vi "clm.build.flow.parse.vi"(11 "Device Flow":T1[](array[typedef])) -> (0 "error out":errorcluster, 3 "Device Conf":T3={"Schedular"={"sched-mode"=enum."Hourly", "sched-pairs"=[]}, "Sensor"={"Input"="ain", "Comparison"=">=", "Setpoint"=0.0}, "Outputs"=[], "Interval"=0, "Timeout"=0, "Mode"=enum."On"} caption="Device Setup" {"Schedular"."sched-pairs"."start" format="%<%H:%M %d/%m>T"; "Schedular"."sched-pairs"."stop" format="%<%H:%M %d/%m>T"; "Timeout" min=1})   [LabVIEW 2024]
uses:
  controls/UiStepBuilder.ctl
  controls/type.step-builder.ctl
  controls/controller.ctl
  controls/sched-cluster.ctl
  controls/UiScheduleTimestamp.ctl
  controls/UiDeviceSensorParams.ctl
  controls/UiDeviceSensorEquality.ctl
  controls/device-mode.ctl
  controls/sched-encoded-cluster.ctl
panel:
  out "length":i32
  out "Device Flow Out":T1[](array[typedef])=[{"Step Function"=enum."LOG-MESSAGE", "ParamString"="SENSOR", "Step Label"="DEVTYPE"}, {"Step Function"=enum."IO-COMPARE-OUT", "ParamString"="ain,>=,15.0,OFF,", "Step Label"="START"}, {"Step Function"=enum."IO-WRITE", "ParamString"="dout1,1:5", "Step Label"="ON"}, {"Step Function"=enum."JUMP", "ParamString"="WAIT", "Step Label"=""}, {"Step Function"=enum."IO-WRITE", "ParamString"="dout1,0:0", "Step Label"="OFF"}, {"Step Function"=enum."DELAY", "ParamString"="10", "Step Label"="WAIT"}, {"Step Function"=enum."JUMP", "ParamString"="START", "Step Label"=""}]
  # "Pulse [sec]"
  # "Period [sec]"
  # "Sensor"
  # "Scheduler"
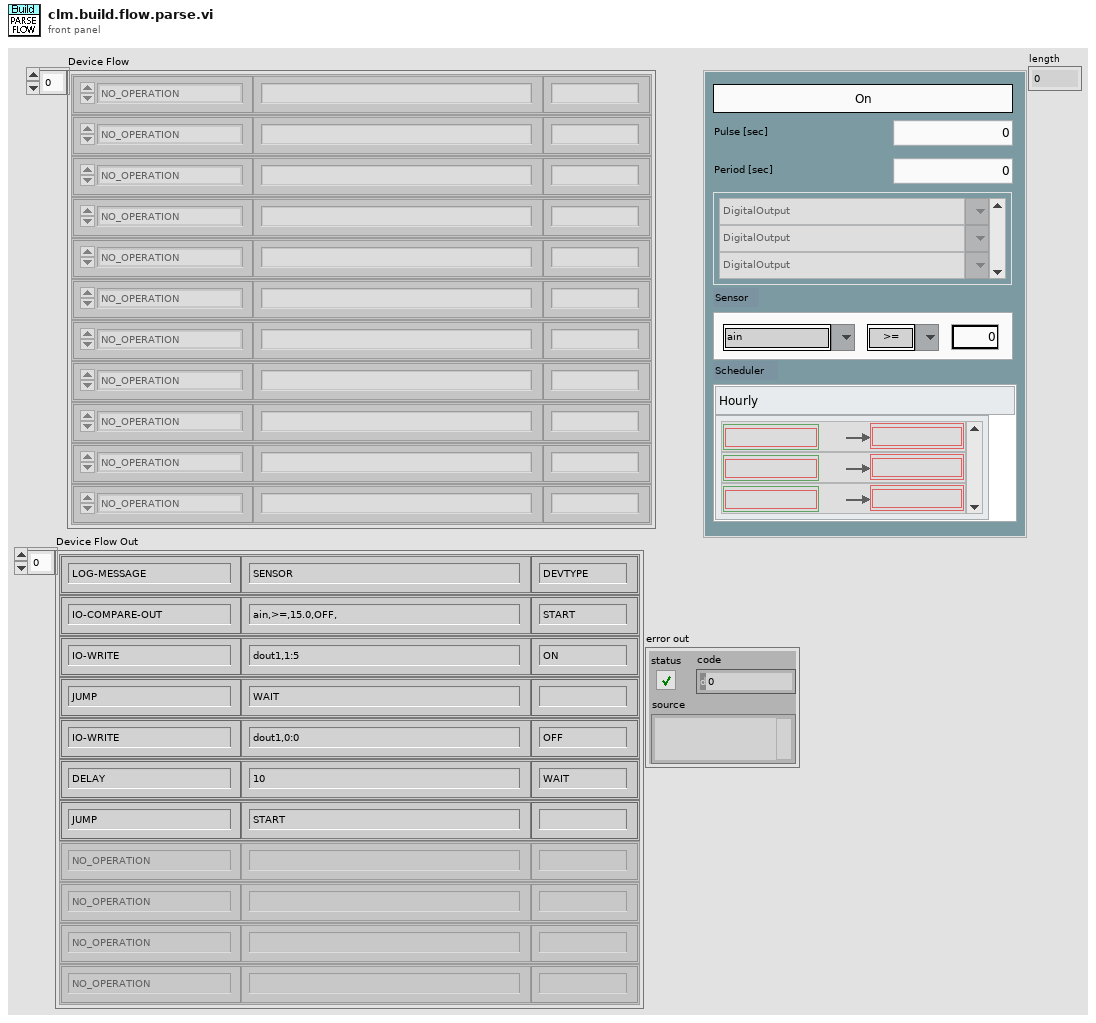
[diagram p1: front panel]
types:
  T1 = typedef "UiStepBuilder.ctl" = cluster{"Step Function":T2, "ParamString":string, "Step Label":string}
  T2 = typedef "type.step-builder.ctl" = enum16{"NO_OPERATION", "DELAY-JUMP", "DELAY", "JUMP", "COMPLETE", "SCHEDULER", "IRR-CHECK", "UNIT-CHECK", "UNIT-SAMPLE", "UNIT-DOSE", "LOG-REPORT", "LOG-MESSAGE", "IO-READ", "IO-READ-MANY", "IO-WRITE", "IO-COMPARE-OUT", "IO-COMPARE-IN", "PROC-START", "PROC-STOP", "PROC-LOAD", "PROC-IS-COMPLETED", "RECORD-MOVE", "GET-RH", "GET-UV", "GET-WD", "GET-WS", "OCS-CHECK", "OCS-RECORD"}
  T3 = typedef "controller.ctl" = cluster{"Schedular":T4, "Sensor":T6, "Outputs":string[], "Interval":u32, "Timeout":u16, "Mode":T8}
  T4 = typedef "sched-cluster.ctl" = cluster{"sched-mode":enum16{"Hourly", "Daily", "Weekly", "Date"}, "sched-pairs":cluster{"start":T5, "stop":T5}[]}
  T5 = typedef "UiScheduleTimestamp.ctl" = timestamp
  T6 = typedef "UiDeviceSensorParams.ctl" = cluster{"Input":string, "Comparison":T7, "Setpoint":dbl}
  T7 = typedef "UiDeviceSensorEquality.ctl" = string
  T8 = typedef "device-mode.ctl" = enum16{"On", "Off", "Sense", "Sched", "Sched AND Sense", "Sched OR Sense"}
  T9 = typedef "sched-encoded-cluster.ctl" = cluster{"StepPtr":string, "SchedPrms":T4}
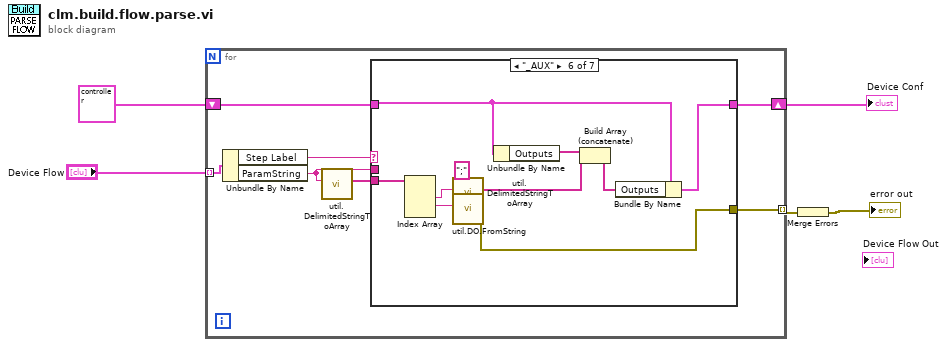
[diagram p0: block diagram]
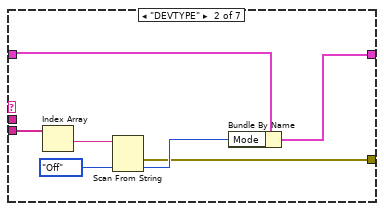
[diagram p3: hidden frame]
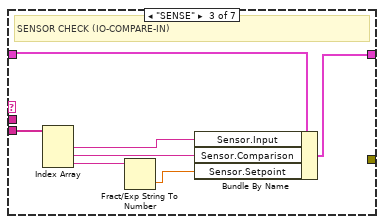
[diagram p4: hidden frame]
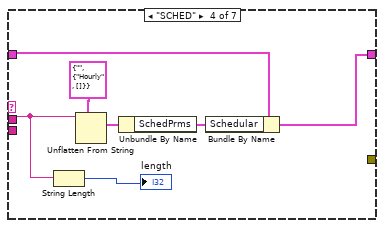
[diagram p5: hidden frame]
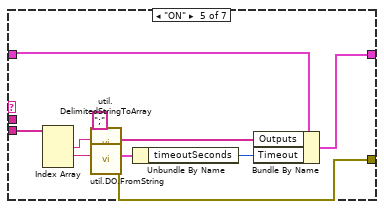
[diagram p6: hidden frame]
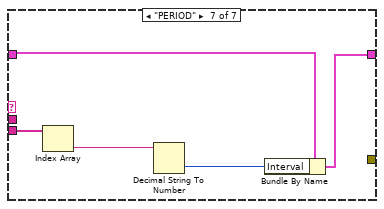
[diagram p7: hidden frame]
diagram:
  n1 = for {
    tunnel: "Device Flow" -> [w12] mode=indexing
    shift-right: [w8] -> w3
    shift-left: T3 {"Schedular"={"sched-mode"=enum."Hourly", "sched-pairs"=[]}, "Sensor"={"Input"="ain", "Comparison"=">=", "Setpoint"=0.0}, "Outputs"=[], "Interval"=0, "Timeout"=0, "Mode"=enum."On"} ("Device") -> [w10]
    tunnel: [w7] -> w1 mode=indexing
    n2 = Unbundle By Name(w12) -> ("Step Label"=w11:string, "ParamString"=w6:string)
    n3 = call "util.DelimitedStringToArray.vi"("delimitaed string"=w6) -> ("array out"=w9:string[])  [unwired: 10 in]
    n4 = case shown="\"_AUX\"" w11 {
      tunnel: w10 -> [w13 w20 w27 w33 w44 w48 w59]
      tunnel: w9 -> [_ w18 w25 _ w42 w53 w57]
      tunnel: [w13 w19 w26 w34 w43 w54 w58] -> w8
      tunnel: [_ w14 _ _ w35 w49 _] -> w7
      tunnel: w6 -> [_ _ _ w29 _ _ _]
      frame Default {
      }
      frame "DEVTYPE" {
        n5 = Index Array(array=w18) -> (element=w17:string)  [unwired: 1 in]
        n6 = Scan From String(input string=w17, default 1=device-mode."Off" ("Mode")) -> (error out=w14:errorcluster, output 1=w15:T8)  [unwired: 3 in, 2 out]
        n7 = Bundle By Name(cluster=w20, "Mode"=w15) -> (w19:T3)
      }
      frame "SENSE" {
        # "SENSOR CHECK (IO-COMPARE-IN)"
        n8 = Index Array(array=w25) -> (element #1=w24:string, element #2=w23:string, element #3=w22:string)  [unwired: 3 in]
        n9 = Fract/Exp String To Number(string=w22) -> (number=w21:dbl)  [unwired: 3 in, 1 out]
        n10 = Bundle By Name(cluster=w27, "Sensor.Input"=w24, "Sensor.Comparison"=w23, "Sensor.Setpoint"=w21) -> (w26:T3)
      }
      frame "SCHED" {
        n11 = String Length(string=w29) -> (length=→"length":i32)
        n12 = Unflatten From String(type=T9 {"StepPtr"="", "SchedPrms"={"sched-mode"=enum."Hourly", "sched-pairs"=[]}} ("cluster"), binary string=w29) -> (value=w32:T9)  [unwired: 3 in, 2 out]
        n13 = Unbundle By Name(w32) -> ("SchedPrms"=w31:T4)
        n14 = Bundle By Name(cluster=w33, "Schedular"=w31) -> (w34:T3)
      }
      frame "ON" {
        n15 = Index Array(array=w42) -> (element #1=w41:string, element #2=w38:string)  [unwired: 3 in, 1 out]
        n16 = call "util.DelimitedStringToArray.vi"("delimiter (,)"=";", "delimitaed string"=w41) -> ("array out"=w40:string[])  [unwired: 9 in]
        n17 = call "util.DO.FromString.vi"("initial string"=w38) -> ("error IO"=w35:errorcluster, "output cluster"=w37:cluster{"state":bool, "timeoutSeconds":u16})  [unwired: 9 in]
        n18 = Unbundle By Name(w37) -> ("timeoutSeconds"=w36:u16)
        n19 = Bundle By Name(cluster=w44, "Outputs"=w40, "Timeout"=w36) -> (w43:T3)
      }
      frame "_AUX" {
        n20 = Index Array(array=w53) -> (element #1=w52:string, element #2=w50:string)  [unwired: 3 in, 1 out]
        n21 = call "util.DelimitedStringToArray.vi"("delimiter (,)"=";", "delimitaed string"=w52) -> ("array out"=w46:string[])  [unwired: 9 in]
        n22 = call "util.DO.FromString.vi"("initial string"=w50) -> ("error IO"=w49:errorcluster)  [unwired: 9 in, 1 out]
        n23 = Unbundle By Name(w48) -> ("Outputs"=w47:string[])
        n24 = Build Array (concatenate)(w47, w46) -> (w45:string[])
        n25 = Bundle By Name(cluster=w48, "Outputs"=w45) -> (w54:T3)
      }
      frame "PERIOD" {
        n26 = Index Array(array=w57) -> (element=w56:string)  [unwired: 1 in]
        n27 = Decimal String To Number(string=w56) -> (number=w55:i32)  [unwired: 2 in, 1 out]
        n28 = Bundle By Name(cluster=w59, "Interval"=w55) -> (w58:T3)
      }
    }
  }
  "Device Conf" <- w3
  n29 = Merge Errors(w1) -> (→"error out":errorcluster)
